vi "Get Parameter String.vi"(8 "error in (no error)":errorcluster, 10 "Exception Names":string[](array[string])=["wait for reply (T)", "error in", "Show Main VI Diagram on Init (F)", "Origin", "Wait for Module to Stop? (F)", "Timeout to Wait for Stop (s) (-1: no timeout)"], 11 "Array":refnum<vi>[](array[refnum])) -> (0 "error out":errorcluster, 3 "parameters":string)   [LabVIEW 2025, in "Scripting Server.lvlib" / "Tools.lvlib"]
uses:
  Tools.lvlib
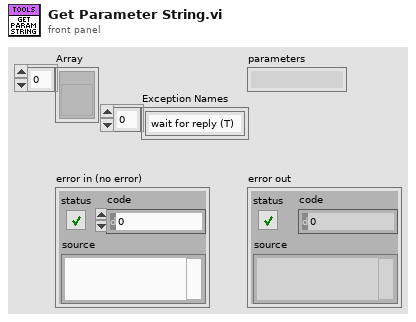
[diagram p1: front panel]
types:
  T1 = typedef "Datatypes.ctl" = enum16{"Float", "Int", "String", "String Array", "Int Array", "Float Array", "Bool Array", "Bool", "Invalid"}
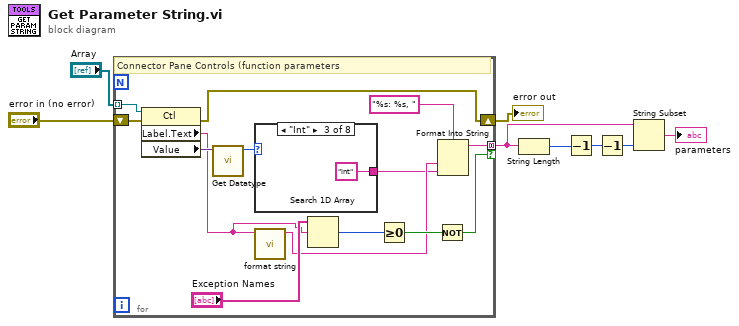
[diagram p0: block diagram]
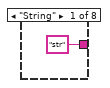
[diagram p2: hidden frame]
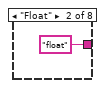
[diagram p3: hidden frame]
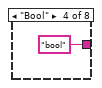
[diagram p4: hidden frame]
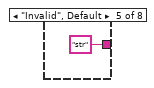
[diagram p5: hidden frame]
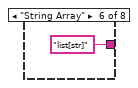
[diagram p6: hidden frame]
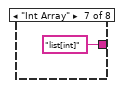
[diagram p7: hidden frame]
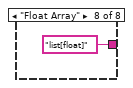
[diagram p8: hidden frame]
diagram:
  n1 = for {
    tunnel: "Array" -> [w20] mode=indexing
    shift-right: [w21] -> w3
    shift-left: "error in (no error)" -> [w22]
    tunnel: [w15] -> w7 mode=concatenating if=w16
    # "Connector Pane Controls (function parameters"
    n2 = property class="Ctl"(reference=w20, error in=w22) -> (error out=w21:errorcluster, "Label.Text"=w9:string, "Value"=w11:variant)  [unwired: 1 out]
    n3 = call "Get Datatype.vi"("Value"=w11) -> ("datatypes"=w12:T1)  [unwired: 10 in]
    n4 = case shown="\"Int\"" w12 {
      tunnel: ["str" ("format string") "float" ("format string") "int" ("format string") "bool" ("format string") "str" ("format string") "list[str]" ("format string") "list[int]" ("format string") "list[float]" ("format string")] -> w10
      frame "String" {
      }
      frame "Float" {
      }
      frame "Int" {
      }
      frame "Bool" {
      }
      frame "Invalid", Default {
      }
      frame "String Array" {
      }
      frame "Int Array" {
      }
      frame "Float Array" {
      }
    }
    n5 = call "format string.vi"("Label.Text"=w9) -> ("String"=w13:string)  [unwired: 10 in]
    n6 = Search 1D Array(1D array="Exception Names", element=w9) -> (index of element=w18:i32)  [unwired: 1 in]
    n7 = Greater Or Equal To 0?(x=w18) -> (x >= 0?=w17:bool)
    n8 = Not(x=w17) -> (.not. x?=w16:bool)
    n9 = Format Into String(format string="%s: %s, ", w13, w10) -> (resulting string=w15:string)  [unwired: 2 in, 1 out]
  }
  "error out" <- w3
  n10 = String Length(string=w7) -> (length=w6:i32)
  n11 = Decrement(x=w6) -> (x-1=w8:i32)
  n12 = Decrement(x=w8) -> (x-1=w5:i32)
  n13 = String Subset(string=w7, length (rest)=w5) -> (substring=→"parameters":string)  [unwired: 1 in]
